vi "sub_Spectrogram.vi"(11 "data":waveform(dbl)) -> (0 "Y Scale.Offset and Multiplier:Multiplier":dbl, 1 "X Scale.Offset and Multiplier:Multiplier":dbl, 2 "X Scale.Range:Maximum":dbl, 3 "STFT Spectrogram":dbl[][](graph), 4 "Z Scale.Marker Values[]":cluster{dbl, u32}[](array[cluster])=[{-1.0, 0}, {-2.0, 16711680}, {-5.0, 16776281}, {-8.0, 16448250}])   [LabVIEW 2014]
doc: "This VI illustrates how to play a sound file continuously, reading the sound file in pieces, and playing each piece at a time. \n------------------------------------\nAuther: Koji Ohashi\nCopyright (c) 2020 Japan LabVIEW Users Group, Volunteer members.\nThis VI is released under the MIT License.\nhttp://opensource.org/licenses/mit-license.php\n------------------------------------"
uses:
  <vilib>/gmath/NI_Gmath.lvlib
  <vilib>/Analysis/4window.llb/windowTd.ctl
  <vilib>/Analysis/NI_AALPro.lvlib
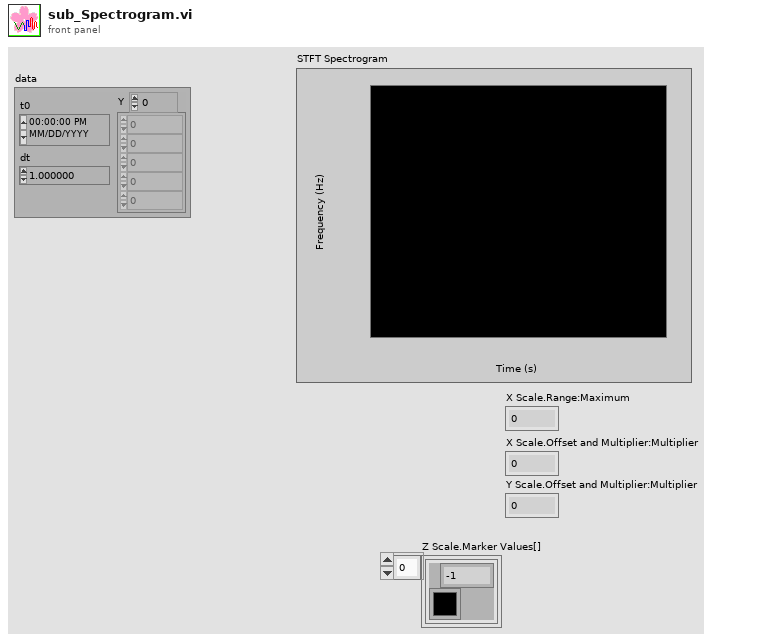
[diagram p1: front panel]
types:
  T1 = typedef "NI_AALPro.lvlib/windowTd.ctl" = u32
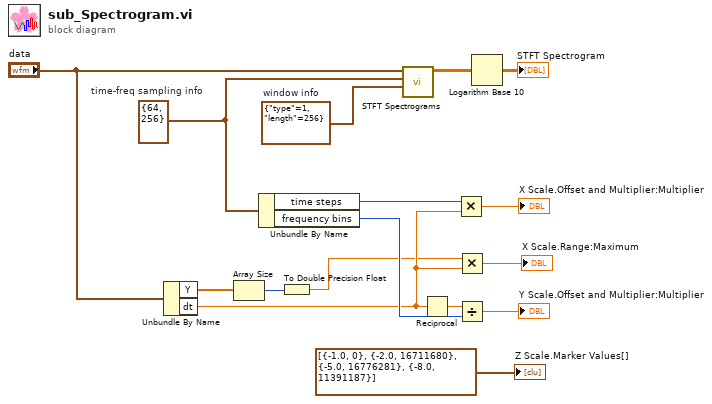
[diagram p0: block diagram]
diagram:
  w14 = cluster{"type":T1, "length":i32} {"type"=1, "length"=256}  # window info
  w13 = cluster{"time steps":i32, "frequency bins":i32} {"time steps"=64, "frequency bins"=256}  # time-freq sampling info
  n1 = Unbundle By Name("data") -> ("Y"=w4:dbl[], "dt"=w5:dbl)
  n2 = Array Size(array=w4) -> (size(s)=w3:i32)
  n3 = Unbundle By Name(w13) -> ("time steps"=w16:i32, "frequency bins"=w15:i32)
  n4 = To Double Precision Float(number=w3) -> (double precision float=w2:dbl)
  n5 = call <vilib>:"STFT Spectrograms.vi"("window info"=w14, "time-freq sampling info"=w13, "X"="data") -> ("STFT Spectrogram {X}"=w10:dbl[][])  [unwired: 3 in, 5 out]
  n6 = Reciprocal(x=w5) -> (1/x=w6:dbl)
  n7 = Multiply(x=w16, y=w5) -> (x*y=→"X Scale.Offset and Multiplier:Multiplier":dbl)
  n8 = Multiply(x=w2, y=w5) -> (x*y=→"X Scale.Range:Maximum":dbl)
  n9 = Divide(x=w6, y=w15) -> (x/y=→"Y Scale.Offset and Multiplier:Multiplier":dbl)
  n10 = Logarithm Base 10(1:w10) -> (0:→"STFT Spectrogram":dbl[][])
  "Z Scale.Marker Values[]" <- cluster{dbl, u32}[] [{-1.0, 0}, {-2.0, 16711680}, {-5.0, 16776281}, {-8.0, 11391187}] ("Z Scale.Marker Values[]")
